vi "New 2ch.vi"(0 "VISA resource name out":refnum<visa-resource-name>, 9 "Number of channels":i32, 11 "error out":errorcluster) -> (3 "VISA resource name out 2":refnum<visa-resource-name>, 4 "Array 2":dbl[](array[numeric]), 6 "Array":dbl[](array[numeric]), 15 "error out 2":errorcluster)   [LabVIEW 2015]
uses:
  <instrlib>/Keithley 27XX/Public/Data/Read Multiple Direct.vi
  <instrlib>/Keithley 27XX/Keithley 27XX.lvlib
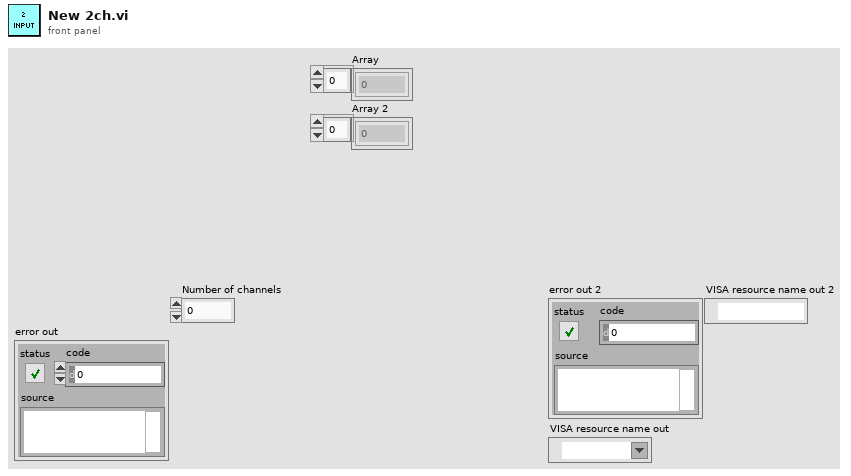
[diagram p1: front panel]
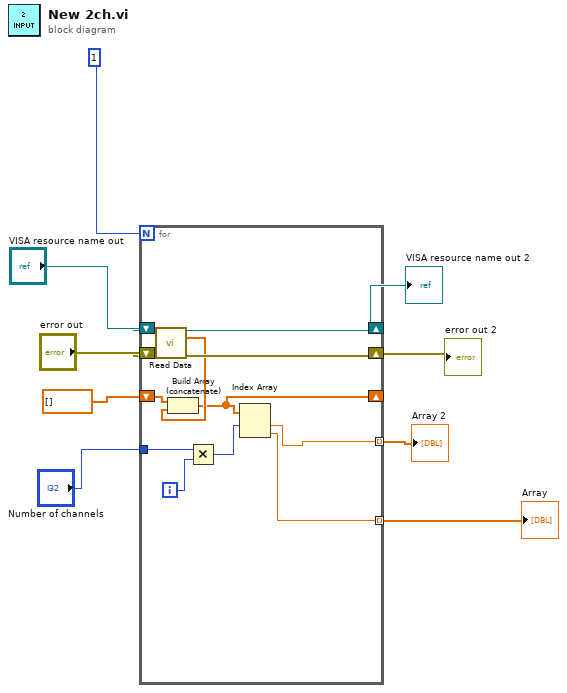
[diagram p0: block diagram]
diagram:
  n1 = for {
    N: 1 -> [_]
    shift-right: [w20] -> w8
    shift-left: "VISA resource name out" -> [w19]
    shift-right: [w21] -> w9
    shift-left: "error out" -> [w18]
    shift-right: [w12] -> _
    shift-left: dbl[] [] -> [w17]
    tunnel: "Number of channels" -> [w14]
    tunnel: [w11] -> w2 mode=indexing
    tunnel: [w10] -> w1 mode=indexing
    i -> [w15]
    n2 = call-poly <instrlib>:"Read Data.vi"("VISA resource name"=w19, "error in (no error)"=w18) -> ("VISA resource name out"=w20:refnum<visa-resource-name>, "Measurement Data"=w16:dbl[], "error out"=w21:errorcluster)  [unwired: 8 in, 3 out]
    n3 = Build Array (concatenate)(w17, w16) -> (w12:dbl[])
    n4 = Multiply(x=w14, y=w15) -> (x*y=w13:i32)
    n5 = Index Array(array=w12, index #1=w13) -> (element #1=w11:dbl, element #2=w10:dbl)  [unwired: 1 in]
  }
  "error out 2" <- w9
  "VISA resource name out 2" <- w8
  "Array" <- w1
  "Array 2" <- w2
